vi "RGBlezen.vi"(2 "error in (no error)":errorcluster) -> (0 "Boolean":bool)   [LabVIEW 2019]
uses:
  <vilib>/myRIO/Instrument Drivers/Onboard IO/I2C/typedefs/I2C User Configuration.ctl
  <vilib>/myRIO/Instrument Drivers/Onboard IO/I2C/typedefs/I2C Transfer Rate.ctl
  <vilib>/myRIO/Instrument Drivers/Onboard IO/I2C/typedefs/I2C Reference.ctl
  <vilib>/myRIO/Common/Instrument Driver Framework/Utilities/typedefs/myRIO Generic Hardware Reference.ctl
  <vilib>/myRIO/Common/Instrument Driver Framework/Utilities/typedefs/Hardware Version Enum.ctl
  <vilib>/myRIO/Common/Instrument Driver Framework/Utilities/typedefs/myRIO v1.0 Reference.ctl
  <vilib>/myRIO/Common/Instrument Driver Framework/Utilities/typedefs/Generic FPGA Reference.ctl
  <vilib>/myRIO/Common/Instrument Driver Framework/myRIO v1.0/I2C/typedefs/I2C Channels Enum.ctl
  <vilib>/myRIO/Instrument Drivers/Onboard IO/I2C/typedefs/I2C Configuration.ctl
  <vilib>/userDefined/High Color/nirio_resource_hc.ctl
  <vilib>/myRIO/Common/Instrument Driver Framework/Utilities/vis/Is FPGA Ref Available.vi
  <vilib>/myRIO/Common/Instrument Driver Framework/myRIO v1.0/I2C/vis/myRIO v1.1 Open I2C.vi
  <vilib>/myRIO/Instrument Drivers/Onboard IO/I2C/vis/Configure.vi
  <vilib>/myRIO/Instrument Drivers/Onboard IO/I2C/vis/Write Read.vi
  <vilib>/myRIO/Common/Instrument Driver Framework/Utilities/vis/Validate Channels.vi
  <vilib>/myRIO/Common/Instrument Driver Framework/myRIO v1.0/I2C/vis/myRIO v1.0 Reserve I2C.vi
  <vilib>/myRIO/Common/Instrument Driver Framework/myRIO v1.0/I2C/vis/myRIO v1.0 Build MUX Configuration I2C.vi
  <vilib>/myRIO/Common/Instrument Driver Framework/myRIO v1.0/Resource Manager/vis/myRIO v1.0 Reserve Channel List.vi
  <vilib>/myRIO/Common/Instrument Driver Framework/myRIO v1.0/Resource Manager/vis/myRIO v1.0 Create Configuration List.vi
  <vilib>/myRIO/Common/Instrument Driver Framework/myRIO v1.0/Resource Manager/vis/myRIO v1.0 Reserve Channel.vi
  <vilib>/myRIO/Common/Instrument Driver Framework/myRIO v1.0/Resource Manager/vis/myRIO v1.0 Unreserve Channel.vi
  <vilib>/myRIO/Common/Instrument Driver Framework/myRIO v1.0/Resource Manager/vis/myRIO v1.0 Build Mutex Name.vi
  <vilib>/Utility/VariantDataType/GetNumericInfo.vi
  <vilib>/Utility/error.llb/Error Cluster From Error Code.vi
  <vilib>/myRIO/Common/Instrument Driver Framework/myRIO v1.0/myRIO v1.1 Open.vi
  <vilib>/myRIO/Common/Instrument Driver Framework/Utilities/vis/IO Manager.vi
  <vilib>/myRIO/Common/Instrument Driver Framework/Utilities/vis/Configuration Manager.vi
  <vilib>/myRIO/Common/Instrument Driver Framework/myRIO v1.0/Resource Manager/vis/myRIO v1.0 Configure IO.vi
  <vilib>/myRIO/Common/Instrument Driver Framework/myRIO v1.0/myRIO v1.0 Close.vi
  <vilib>/myRIO/Common/Instrument Driver Framework/myRIO v1.0/I2C/vis/myRIO v1.0 Configure I2C.vi
  <vilib>/myRIO/Common/Instrument Driver Framework/myRIO v1.0/I2C/vis/myRIO v1.0 Write I2C.vi
  <vilib>/myRIO/Common/Instrument Driver Framework/myRIO v1.0/I2C/vis/myRIO v1.0 Read I2C.vi
  <vilib>/myRIO/Express VI/Onboard IO/I2C/I2C Express VI.xnode
  <vilib>/myRIO/Instrument Drivers/Onboard IO/I2C/vis/myRIO I2C Open.xnode
  <vilib>/myRIO/Instrument Drivers/Onboard IO/I2C/I2C.lvlib
  <vilib>/gmath/NI_Gmath.lvlib
panel:
  out "Array 3":u32[](array[numeric])
  out "x+y":u32
  out "juiste waarden":u32[](array[numeric])
  out "Array 2":i32[](array[numeric])
  out "Array":dbl[](array[numeric])
  out "spread value":dbl
  in  "stop":bool
  in  "High":string="—"
  in  "Low":string="–"
  out "error out 2":errorcluster
  out "Low 2":u8[](array[numeric])
  out "High 2":u8[](array[numeric])
  # "RED: 96, 97"
  # "GREEN: 98, 99"
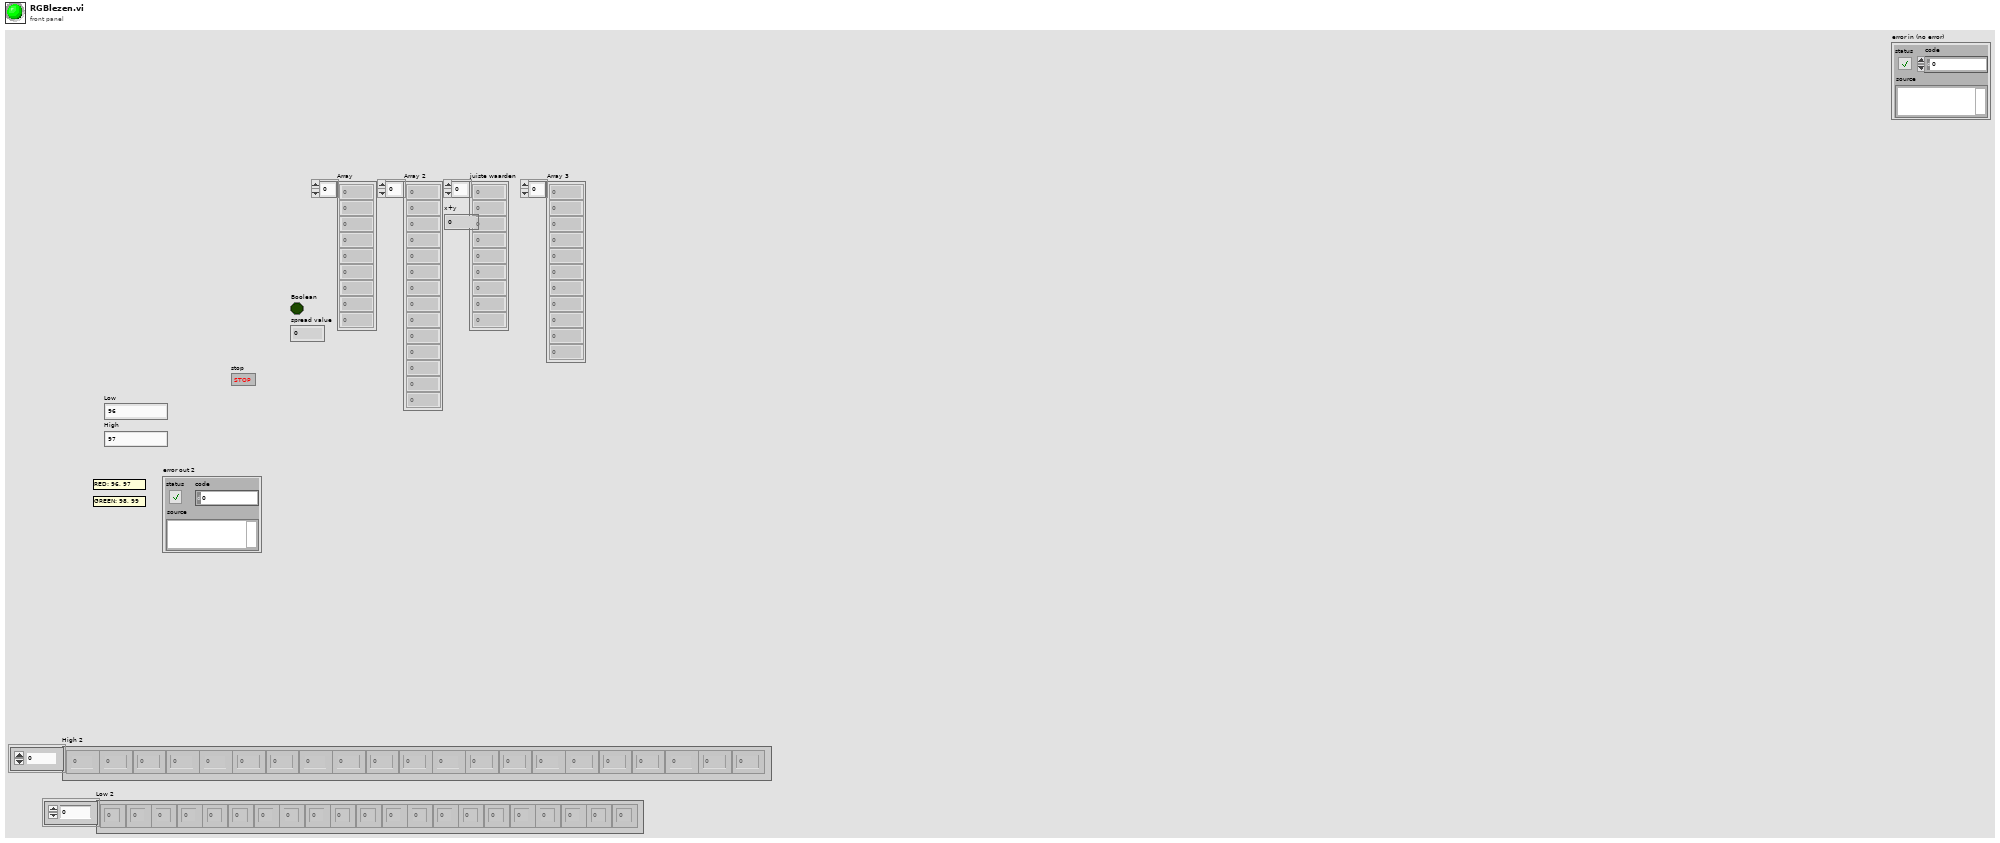
[diagram p1: front panel]
types:
  T1 = typedef "I2C.lvlib/I2C Reference.ctl" = cluster{"myRIO Reference":T2, "I2C Channels Enum":T6, "I2C Configuration":T7}
  T2 = typedef "myRIO Generic Hardware Reference.ctl" = cluster{"myRIO Model":T3, "myRIO Hardware Reference":T4}
  T3 = typedef "Hardware Version Enum.ctl" = enum16{"Unknown", "myRIO-1900", "myRIO-1950", "roboRIO", "NI ELVIS RIO CM", "ELVIS III"}
  T4 = typedef "myRIO v1.0 Reference.ctl" = cluster{"Generic FPGA Reference":T5, "Allow multiple opens":bool}
  T5 = typedef "Generic FPGA Reference.ctl" = refnum<k20>
  T6 = typedef "I2C Channels Enum.ctl" = enum16{"Not Connected", "A/I2C", "B/I2C", "I2C/I2C"}
  T7 = typedef "I2C.lvlib/I2C Configuration.ctl" = cluster{"I2C Transfer Rate":T8}
  T8 = typedef "I2C.lvlib/I2C Transfer Rate.ctl" = enum16{"Standard mode (100 kbps)", "Fast mode (400 kbps)"}
  T9 = typedef "I2C.lvlib/I2C User Configuration.ctl" = cluster{"I2C Transfer Rate":T8}
  T10 = typedef "nirio_resource_hc.ctl" = tag
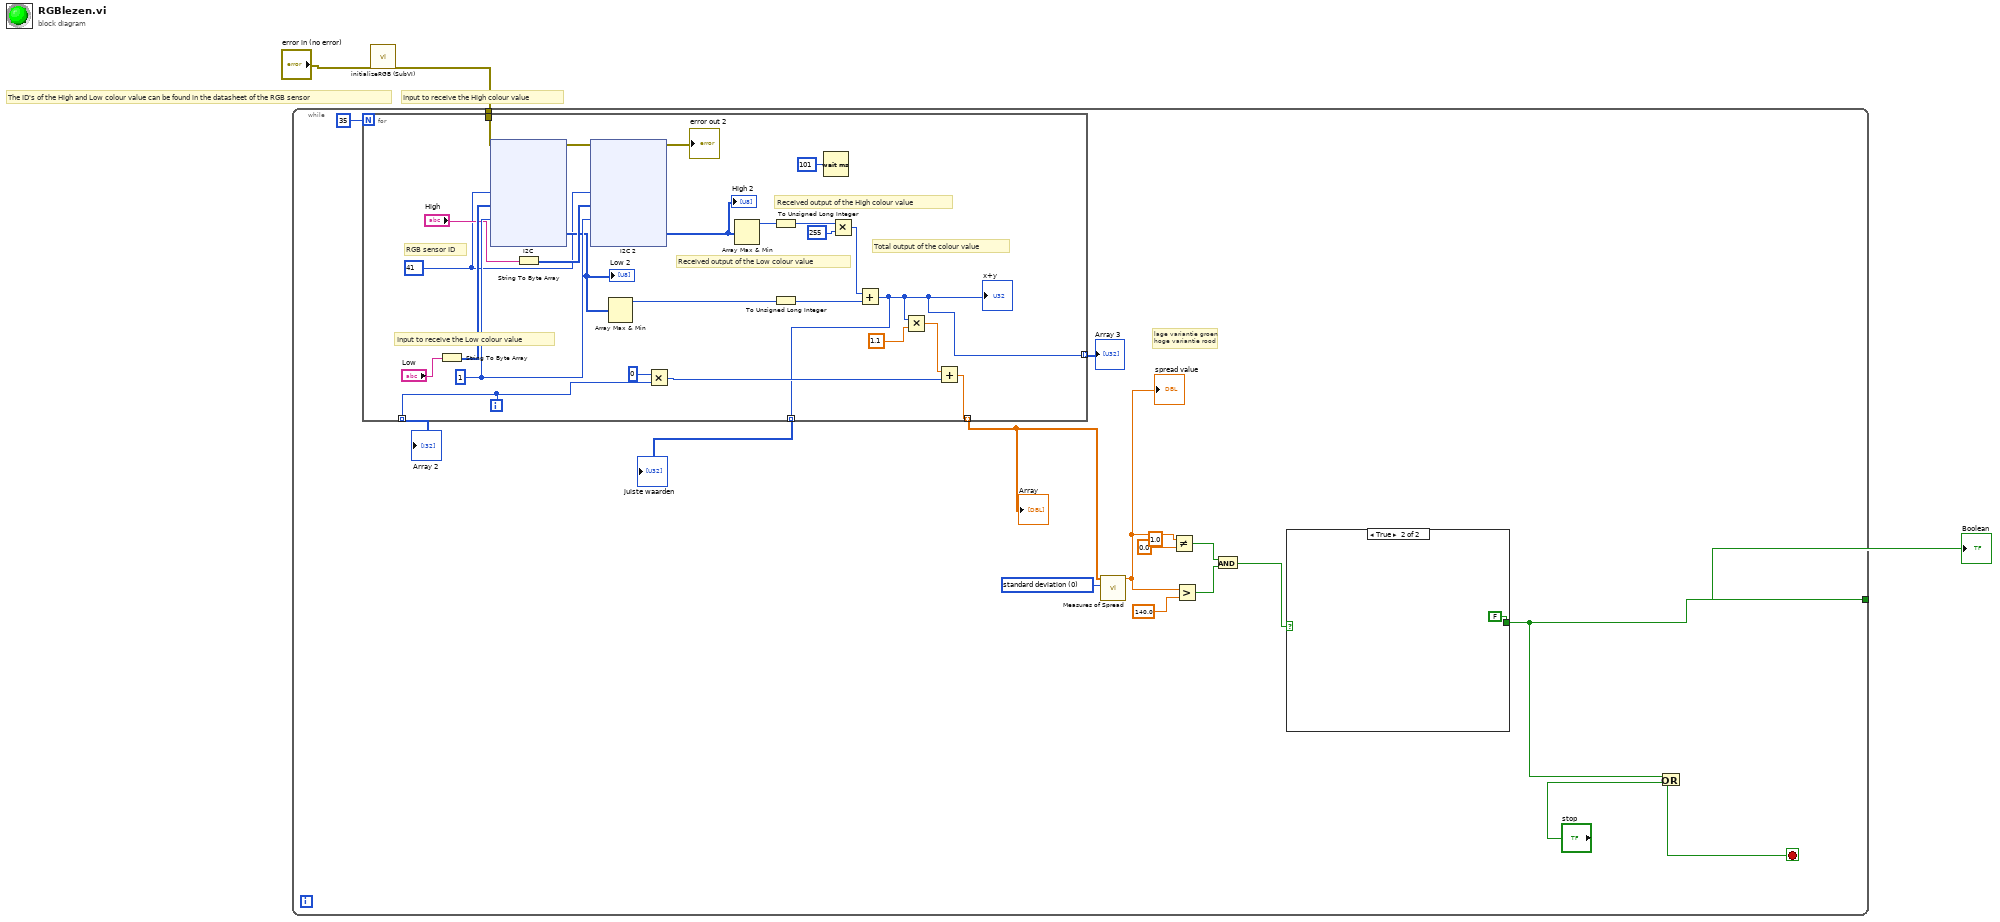
[diagram p0: block diagram]
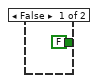
[diagram p2: hidden frame]
diagram:
  # "The ID's of the High and Low colour value can be found in the datasheet of the RGB sensor"
  # "Input to receive the High colour value"
  n1 = call "initializeRGB (SubVI).vi"("error in (no error)"="error in (no error)") -> ("error out"=w2:errorcluster)  [unwired: 10 in]
  n2 = while {
    tunnel: w2 -> [w19]
    tunnel: [w15] -> w1
    stop <- w14 stop-if-true
    (unwired) 1.0 ("x")
    w18 = 0 items=["standard deviation", "range", "mean absolute deviation", "interquartile range"] ("type")
    # "lage variantie groen\nhoge variantie rood"
    n3 = for {
      N: 35 -> [_]
      tunnel: w19 -> [w28]
      tunnel: [w26] -> w7 mode=indexing
      tunnel: [w22] -> w6 mode=indexing
      tunnel: [w21] -> w5 mode=indexing
      tunnel: [w21] -> w4 mode=indexing
      i -> [w26]
      w29 = 41 ("Numeric")
      w41 = u32 1 ("Byte Count")
      # "Total output of the colour value"
      # "Received output of the Low colour value"
      # "Received output of the High colour value"
      # "Input to receive the Low colour value"
      # "RGB sensor ID"
      n4 = String To Byte Array(string="Low") -> (unsigned byte array=w40:u8[])
      n5 = xnode "I2C"("Slave Address (7-bit)"=w29, "Bytes to Write"=w40, "Byte Count"=w41, "error in (no error)"=w28) -> ("Bytes Read"=w37:u8[], "error out"=w42:errorcluster)
      "Low 2" <- w37
      n6 = String To Byte Array(string="High") -> (unsigned byte array=w39:u8[])
      n7 = xnode "I2C 2"("Slave Address (7-bit)"=w29, "Bytes to Write"=w39, "Byte Count"=w41, "error in (no error)"=w42) -> ("Bytes Read"=w36:u8[], "error out"=→"error out 2":errorcluster)
      "High 2" <- w36
      n8 = Array Max & Min(array=w37) -> (max value=w31:u8)  [unwired: 3 out]
      n9 = Multiply(x=0, y=w26) -> (x*y=w24:i32)
      n10 = Array Max & Min(array=w36) -> (max value=w33:u8)  [unwired: 3 out]
      n11 = To Unsigned Long Integer(number=w33) -> (unsigned 32bit integer=w32:u32)
      n12 = To Unsigned Long Integer(number=w31) -> (unsigned 32bit integer=w30:u32)
      n13 = Wait (ms)(milliseconds to wait=u32 101) -> ()  [unwired: 1 out]
      n14 = Multiply(x=w32, y=u32 255) -> (x*y=w34:u32)
      n15 = Add(x=w34, y=w30) -> (x+y=w21:u32)
      "x+y" <- w21
      n16 = Multiply(x=w21, y=1.1) -> (x*y=w23:dbl)
      n17 = Add(x=w23, y=w24) -> (x+y=w22:dbl)
    }
    "Array" <- w6
    "Array 2" <- w7
    "juiste waarden" <- w5
    "Array 3" <- w4
    n18 = call <vilib>:"Measures of Spread.vi"("type"=w18, "x array"=w6) -> ("spread value"=w12:dbl)  [unwired: 8 in, 1 out]
    "spread value" <- w12
    n19 = Not Equal?(x=w12, y=0.0) -> (x != y?=w10:bool)
    n20 = Greater?(x=w12, y=140.0) -> (0:w9:bool)
    n21 = And(x=w10, y=w9) -> (x .and. y?=w8:bool)
    n22 = case shown="True" w8 {
      tunnel: [FALSE FALSE] -> w15
      frame False {
      }
      frame True {
      }
    }
    n23 = Or(x=w15, y="stop") -> (x .or. y?=w14:bool)
  }
  "Boolean" <- w1
